vi "simx Read Force Sensor.vi"(0 "clientID":i32, 1 "torqueVector":sgl, 5 "forceSensorHandle":i32, 7 "state":string, 9 "forceVector":sgl, 11 "error in (no error)":errorcluster, 12 "operationMode":i32) -> (3 "torqueVector out":sgl, 4 "function return":i32, 8 "state out":string, 10 "forceVector out":sgl, 15 "error out":errorcluster)   [LabVIEW 2019, in "PXL_V-REP.lvlib"]
doc: "EXTAPI_DLLEXPORT simxInt simxReadForceSensor(simxInt clientID,simxInt forceSensorHandle,simxUChar* state,simxFloat* forceVector,simxFloat* torqueVector,simxInt operationMode);"
uses:
  PXL_V-REP.lvlib
  <userlib>/V-REP/remoteApi.dll
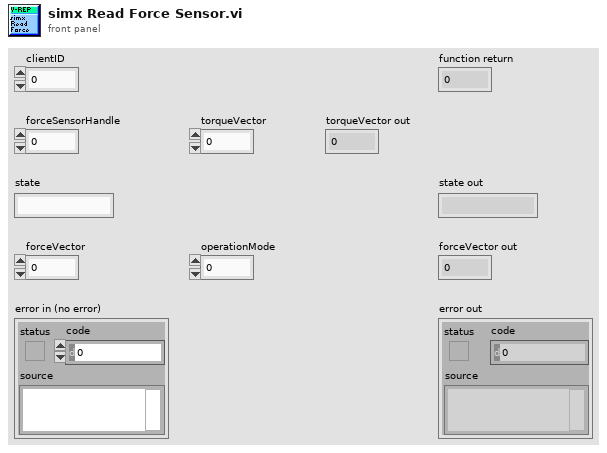
[diagram p1: front panel]
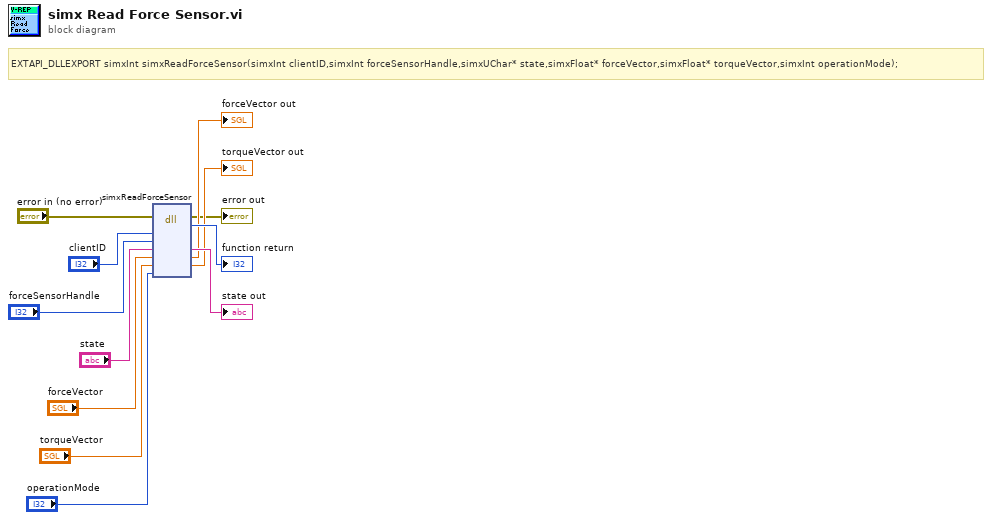
[diagram p0: block diagram]
diagram:
  # "EXTAPI_DLLEXPORT simxInt simxReadForceSensor(simxInt clientID,simxInt forceSensorHandle,simxUChar* state,simxFloat* forceVector,simxFloat* torqueVector,simxInt operationMode);"
  n1 = dll-call lib="C:/Program Files (x86)/National Instruments/LabVIEW 2019/user.lib/V-REP/remoteApi.*" fn="simxReadForceSensor"(error in="error in (no error)", "clientID"="clientID", "forceSensorHandle"="forceSensorHandle", "state"="state", "forceVector"="forceVector", "torqueVector"="torqueVector", "operationMode"="operationMode") -> (error out=→"error out":errorcluster, →"function return":i32, "state"=→"state out":string, "forceVector"=→"forceVector out":sgl, "torqueVector"=→"torqueVector out":sgl)  [unwired: 5 in, 1 out]
